vi "Read_SettingFile_ini.vi"(4 "error in":errorcluster caption="에러 입력(에러 없음)", 7 "Root of Setting File":path) -> (0 "error out":errorcluster caption="에러 출력", 3 "Settings":T1(array[cluster]))   [LabVIEW 2014]
uses:
  <vilib>/Utility/config.llb/Read Key (String).vi
  <vilib>/Utility/config.llb/NI_LVConfig.lvlib
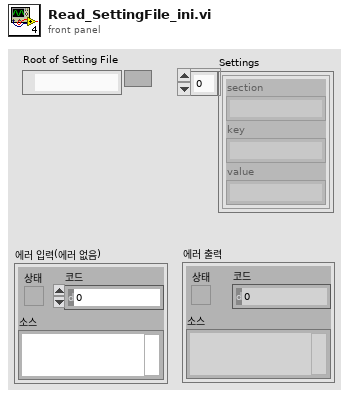
[diagram p1: front panel]
types:
  T1 = cluster{"section":string, "key":string, "value":string}[]
  T2 = typedef "NI_LVConfig.lvlib/Config Data RefNum.ctl" = refnum<k1>
  T3 = cluster{"section":string, "key":string, "value":string}
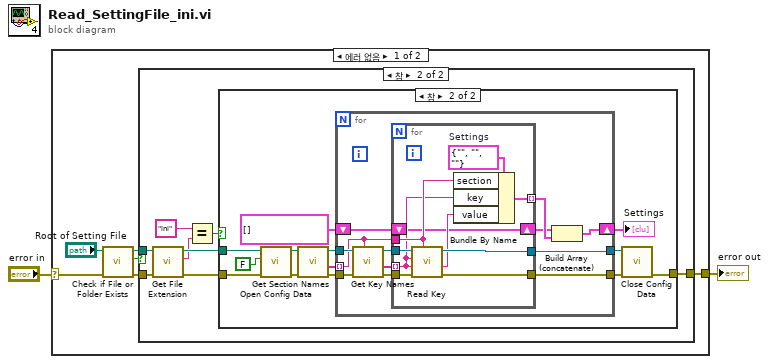
[diagram p0: block diagram]
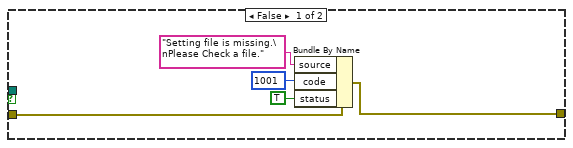
[diagram p2: hidden frame]
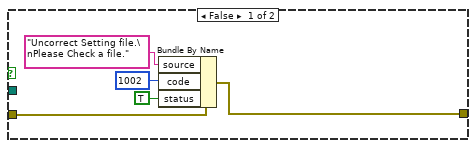
[diagram p3: hidden frame]
diagram:
  n1 = case shown="에러 없음" "error in" {
    selector: "error in" -> [w7 w62]
    tunnel: [w3 w62] -> w1
    frame No Error {
      n2 = call <vilib>:"Check if File or Folder Exists.vi"("error in (no error)"=w7, "path"="Root of Setting File") -> ("error out"=w5:errorcluster, "file or folder exists?"=w6:bool, "dup path"=w4:path)  [unwired: 7 in]
      n3 = case shown="참" w6 {
        tunnel: w5 -> [w10 w17]
        tunnel: w4 -> [_ w18]
        tunnel: [w9 w19] -> w3
        frame False {
          n4 = Bundle By Name(cluster=w10, "source"="Setting file is missing.\nPlease Check a file.", "code"=1001, "status"=TRUE) -> (w9:errorcluster)
        }
        frame True {
          n5 = call <vilib>:"Get File Extension.vi"("error in (no error)"=w17, "file"=w18) -> ("error out"=w16:errorcluster, "lowercase file extension"=w14:string, "dup file"=w15:path)  [unwired: 6 in, 1 out]
          n6 = Equal?(x="ini" ("이후 부분 문자열"), y=w14) -> (x = y?=w20:bool)
          n7 = case shown="참" w20 {
            tunnel: w16 -> [w26 w38]
            tunnel: [w22 w28] -> w19
            tunnel: w15 -> [_ w39]
            frame False {
              n8 = Bundle By Name(cluster=w26, "source"="Uncorrect Setting file.\nPlease Check a file.", "code"=1002, "status"=TRUE) -> (w22:errorcluster)
            }
            frame True {
              n9 = call <vilib>:"Open Config Data.vi"("error in (no error)"=w38, "create file if necessary (T)"=FALSE, "configuration file path"=w39) -> ("error out"=w35:errorcluster, "refnum"=w36:T2)  [unwired: 6 in, 1 out]
              n10 = call <vilib>:"Get Section Names.vi"("error in (no error)"=w35, "refnum"=w36) -> ("error out"=w33:errorcluster, "section names"=w32:string[], "refnum out"=w34:T2)  [unwired: 7 in]
              n11 = for {
                tunnel: w34 -> [w50]
                tunnel: w33 -> [w51]
                tunnel: w32 -> [w49] mode=indexing
                shift-right: [w42] -> w27
                shift-left: T1 [] -> [w44]
                tunnel: [w41] -> w29
                tunnel: [w40] -> w30
                n12 = call <vilib>:"Get Key Names.vi"("section"=w49, "error in (no error)"=w51, "refnum"=w50) -> ("error out"=w47:errorcluster, "key names"=w46:string[], "refnum out"=w48:T2)  [unwired: 5 in, 1 out]
                n13 = for {
                  tunnel: w49 -> [w56]
                  tunnel: w48 -> [w60]
                  tunnel: w47 -> [w61]
                  tunnel: w46 -> [w55] mode=indexing
                  tunnel: [w59] -> w41
                  tunnel: [w58] -> w40
                  tunnel: [w53] -> w45 mode=indexing
                  shift-right: [w52] -> w43
                  shift-left: w44 -> [w52]
                  w57 = T3 {"section"="", "key"="", "value"=""}  # Settings
                  n14 = call-poly <vilib>:"Read Key.vi"("section"=w56, "error in (no error)"=w61, "default value"=w55, "key"=w55, "refnum"=w60) -> ("error out"=w58:errorcluster, "value"=w54:string, "refnum out"=w59:T2)  [unwired: 3 in, 1 out]
                  n15 = Bundle By Name(cluster=w57, "section"=w56, "key"=w55, "value"=w54) -> (w53:T3)
                }
                n16 = Build Array (concatenate)(w43, w45) -> (w42:T1)
              }
              "Settings" <- w27
              n17 = call <vilib>:"Close Config Data.vi"("error in (no error)"=w30, "refnum"=w29) -> ("error out"=w28:errorcluster)  [unwired: 8 in, 1 out]
            }
          }
        }
      }
    }
    frame Error {
      # ">> LabVIEW Error >>"
    }
  }
  "error out" <- w1
